vi "FTP Move files.vi"(0 "File Management":T2, 1 "Unmanaged Files Queue":refnum<queue>, 3 "FTP Creds":T1 {"FTP Timeout (S)" min=0 max=300 step=1}, 4 "File output directories":T3={"Archive Location"=path "", "Archive Location 2"=path "<Not A Path>", "OutPut Path"=path "", "Directory(s) To Scan Files"=[]}, 5 "Unmanaged Files prior errors":errorcluster, 6 "Timing true or false to zip files":bool) -> (15 "Unmanaged Files Queue out":refnum<queue>, 16 "Unmanaged files queue error out":errorcluster, 19 "Log file write error condition":errorcluster)   [LabVIEW 2011]
uses:
  Controls/File Path directories.ctl
  Controls/File Management.ctl
  Controls/FTP Credintials.ctl
  <vilib>/Utility/sysdir.llb/System Directory Type.ctl
panel:
  # "File Handling Method"
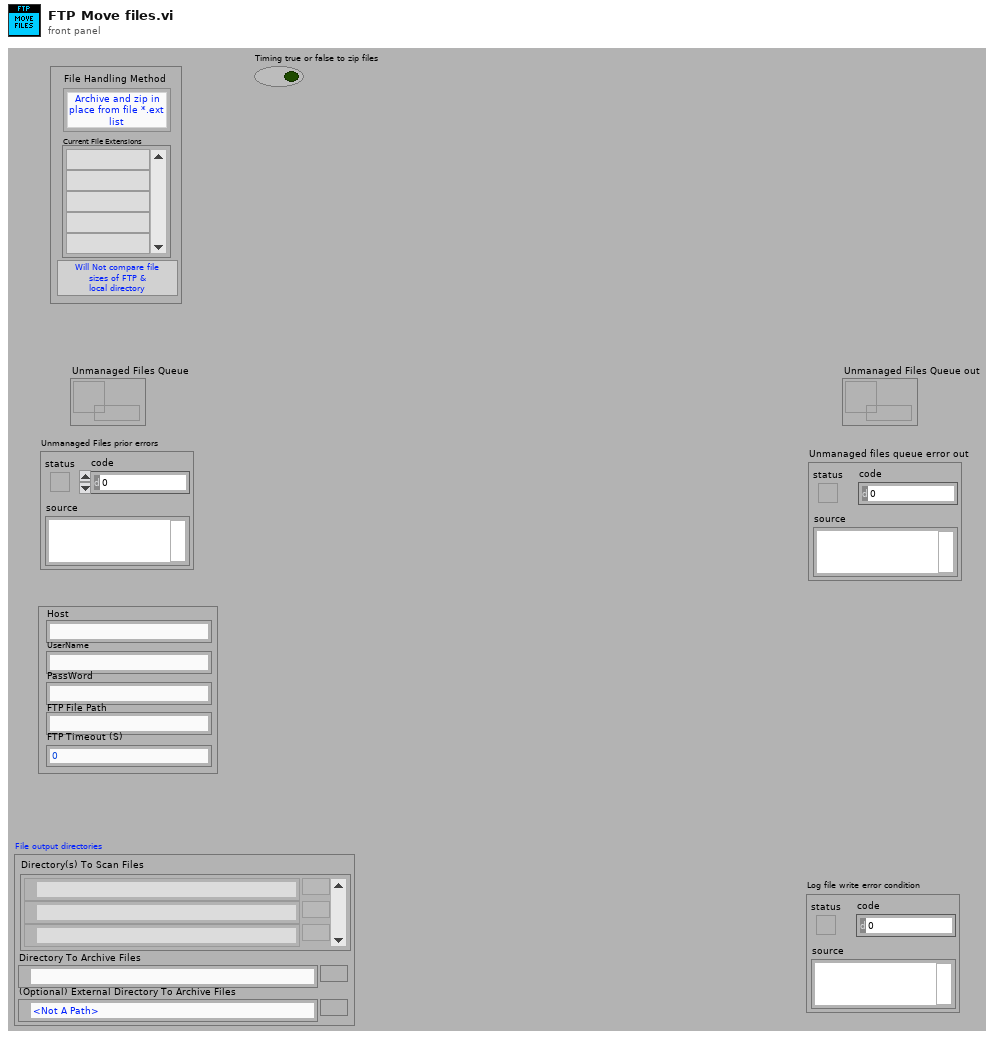
[diagram p1: front panel]
types:
  T1 = typedef "FTP Credintials.ctl" = cluster{"Host":string, "UserName":string, "PassWord":string, "FTP File Path":string, "FTP Timeout (S)":i32, "Active or Passive":bool, "ASCII or Binary":bool}
  T2 = typedef "File Management.ctl" = cluster{"Comp File Size":bool, "File Handle Method":enum16{"Archive and zip in place from file *.ext list", "Archive and zip ALL file Types to archive directory", "Archive and zip to archive directory from file *.ext list", "Perform no file management"}, "file extention list":string[]}
  T3 = typedef "File Path directories.ctl" = cluster{"Archive Location":path, "Archive Location 2":path, "OutPut Path":path, "Directory(s) To Scan Files":path[]}
  T4 = enum16{"Archive and zip in place from file *.ext list", "Archive and zip ALL file Types to archive directory", "Archive and zip to archive directory from file *.ext list", "Perform no file management"}
  T5 = typedef "System Directory Type.ctl" = i32
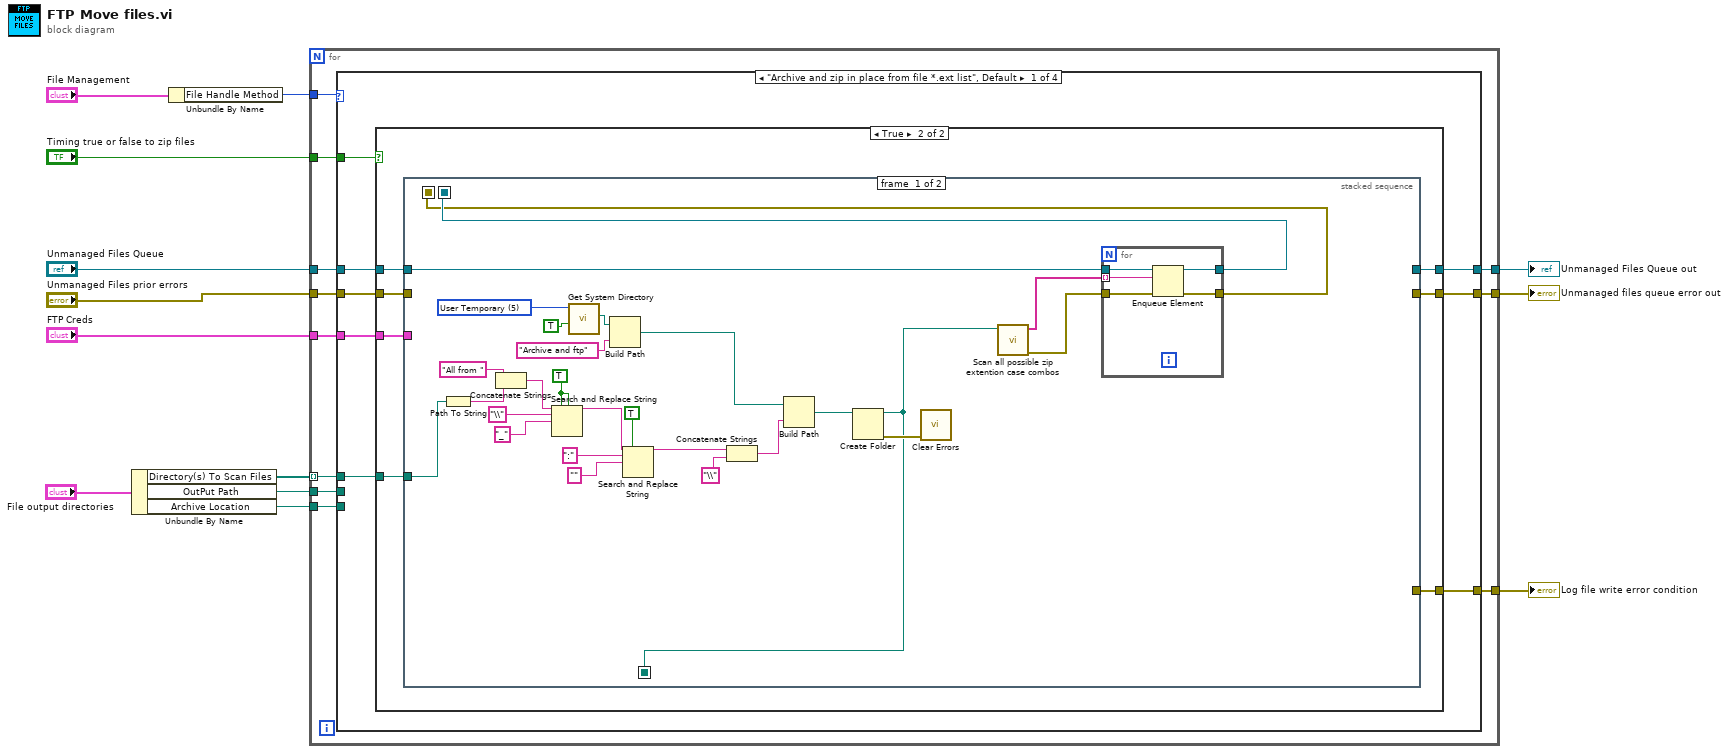
[diagram p0: block diagram]
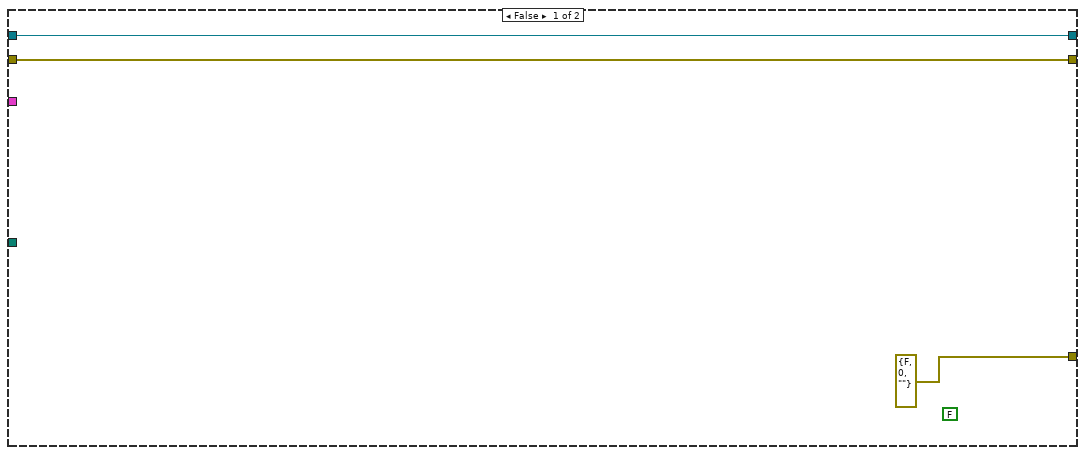
[diagram p2: hidden frame]
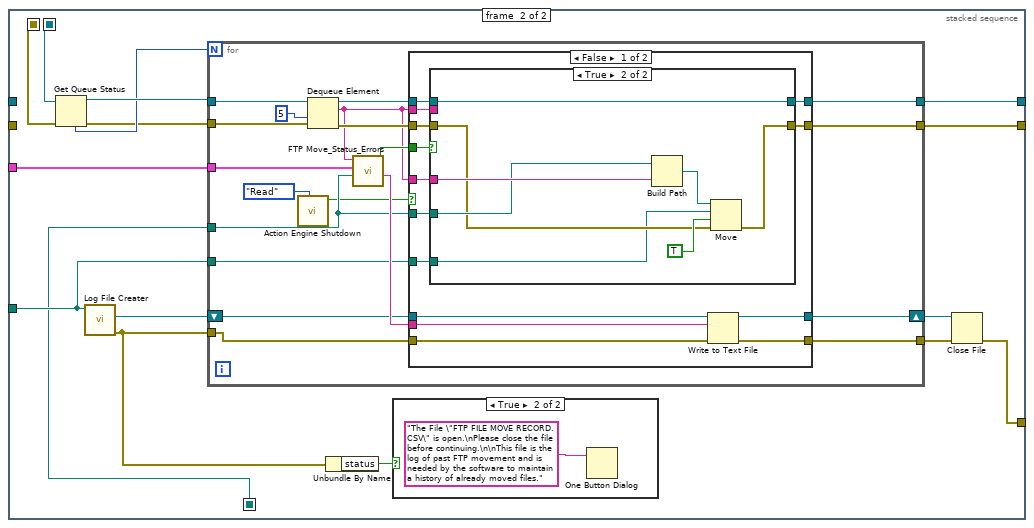
[diagram p3: hidden frame]
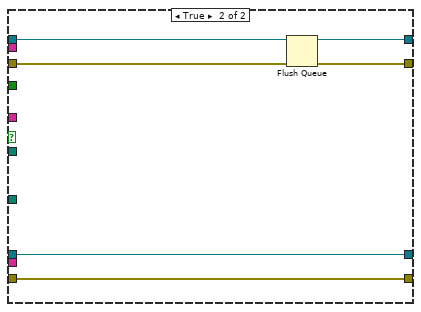
[diagram p6: hidden frame]
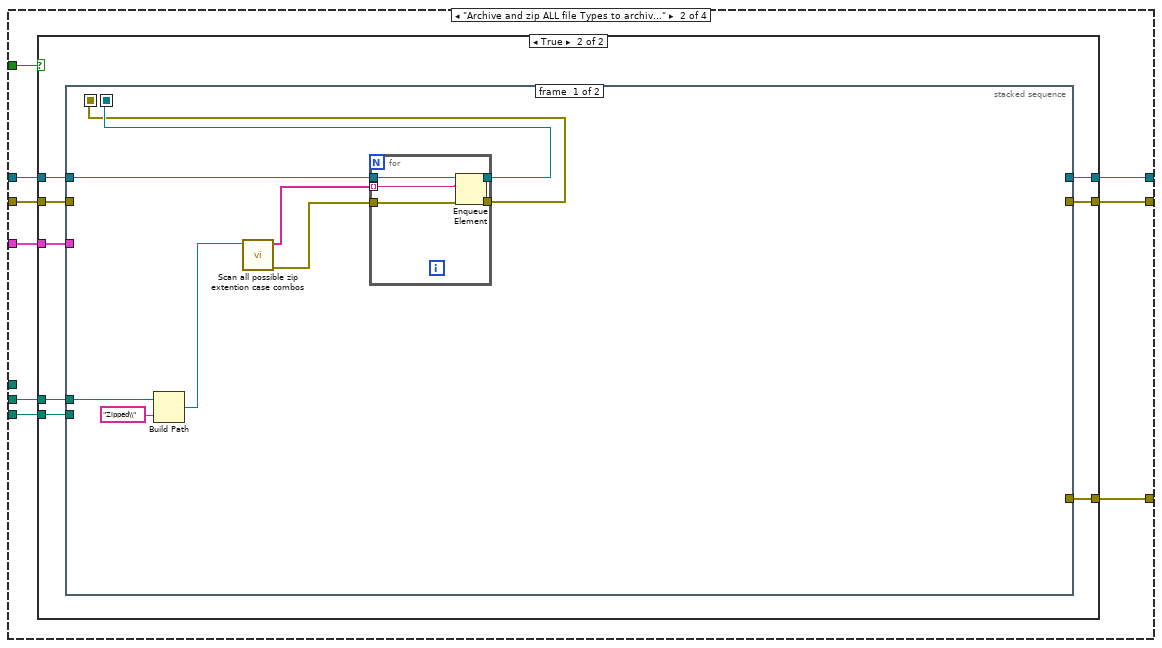
[diagram p7: hidden frame]
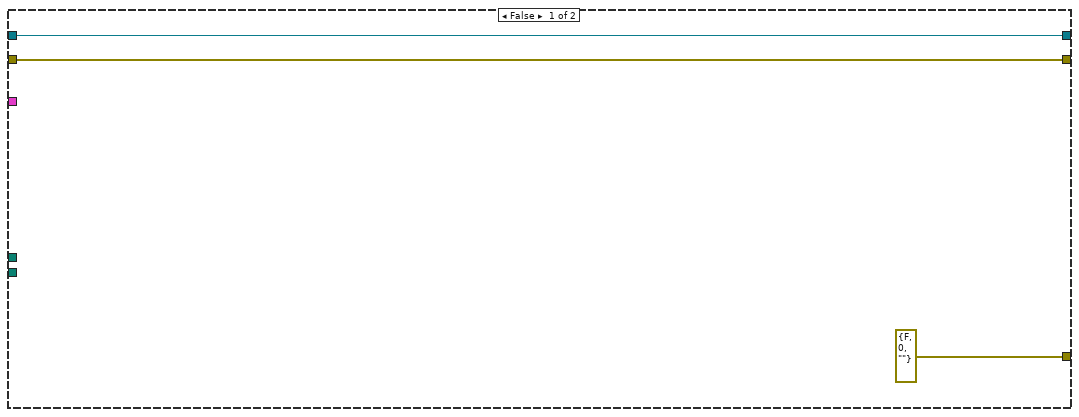
[diagram p8: hidden frame]
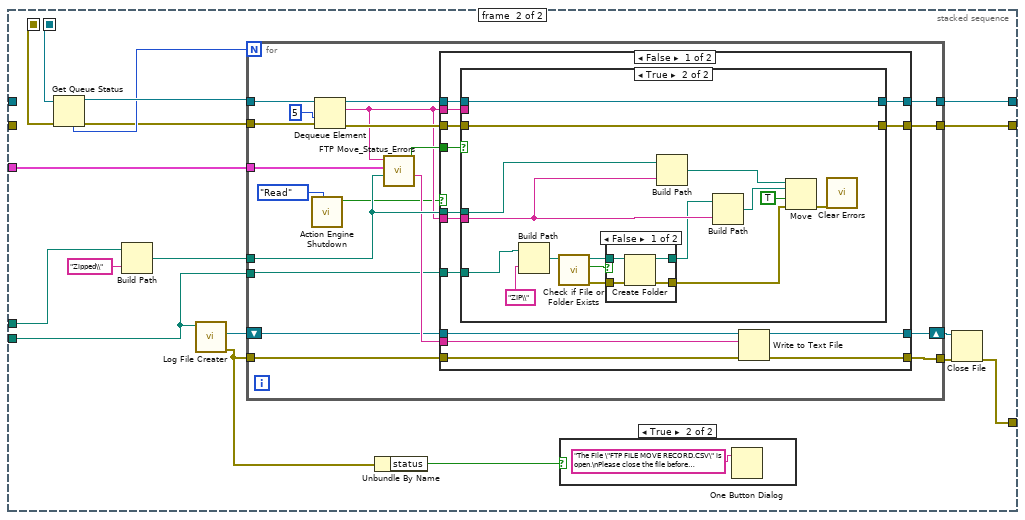
[diagram p9: hidden frame]
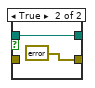
[diagram p12: hidden frame]
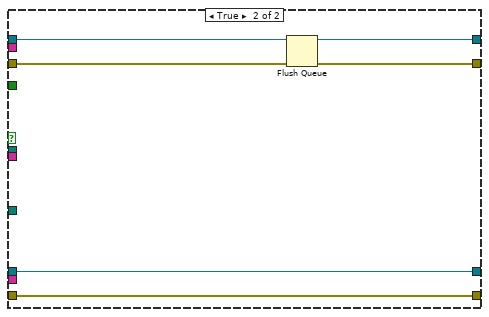
[diagram p13: hidden frame]
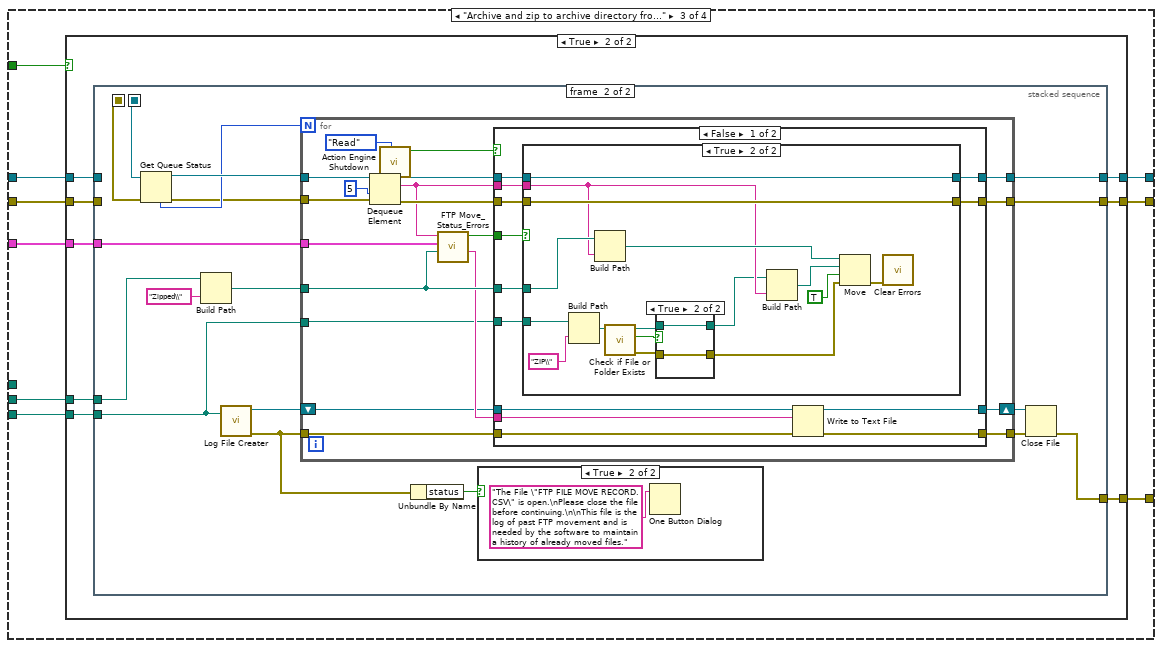
[diagram p14: hidden frame]
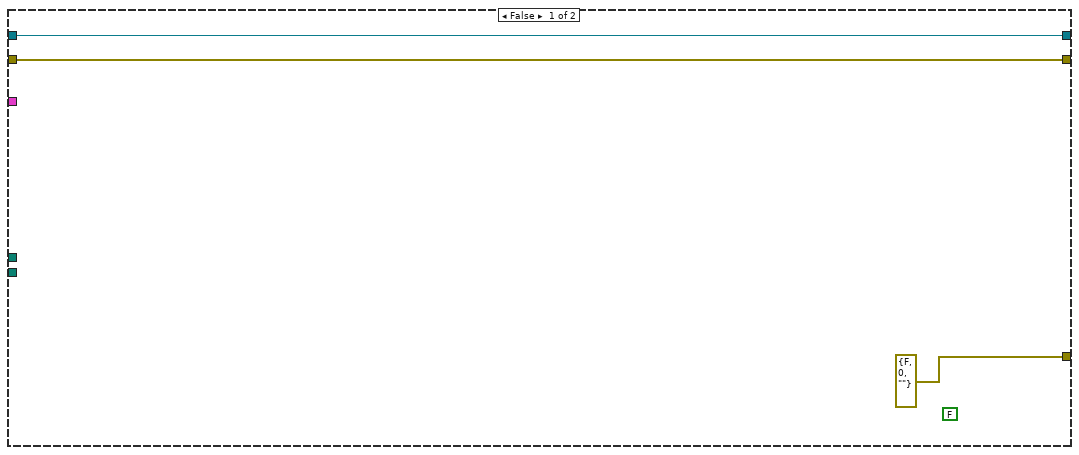
[diagram p15: hidden frame]
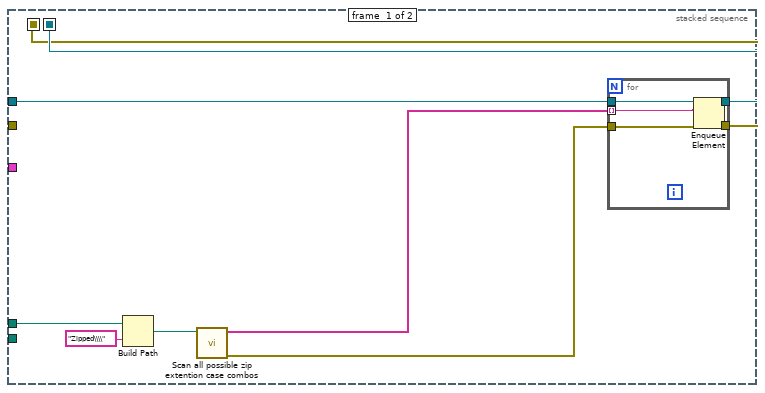
[diagram p16: hidden frame]
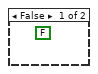
[diagram p17: hidden frame]
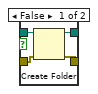
[diagram p19: hidden frame]
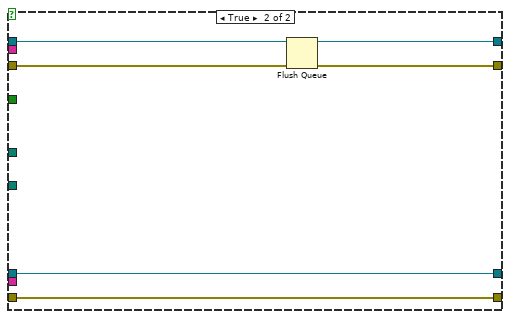
[diagram p20: hidden frame]
diagram:
  n1 = Unbundle By Name("File output directories") -> ("Directory(s) To Scan Files"=w1:path[], "OutPut Path"=w4:path, "Archive Location"=w3:path)
  n2 = Unbundle By Name("File Management") -> ("File Handle Method"=w5:T4)
  n3 = for {
    tunnel: "Unmanaged Files Queue" -> [w24]
    tunnel: "Unmanaged Files prior errors" -> [w23]
    tunnel: "Timing true or false to zip files" -> [w22]
    tunnel: [w21] -> w10
    tunnel: [w20] -> w9
    tunnel: [w19] -> w8
    tunnel: w5 -> [w18]
    tunnel: w4 -> [w17]
    tunnel: w3 -> [w16]
    tunnel: "FTP Creds" -> [w15]
    tunnel: w1 -> [w14] mode=indexing
    n4 = case shown="\"Archive and zip in place from file *.ext list\", Default" w18 {
      tunnel: w24 -> [w31 w149 w263 w372]
      tunnel: w23 -> [w30 w148 w262 w371]
      tunnel: w15 -> [w29 w147 w261 _]
      tunnel: w17 -> [_ w146 w260 _]
      tunnel: w22 -> [w32 w145 w264 _]
      tunnel: [w27 w144 w258 w372] -> w21
      tunnel: [w26 w143 w257 w371] -> w20
      tunnel: [w25 w142 w256 errorcluster {"status"=FALSE, "code"=0, "source"=""} ("error out")] -> w19
      tunnel: w16 -> [_ w141 w259 _]
      tunnel: w14 -> [w28 _ _ _]
      frame "Archive and zip in place from file *.ext list", Default {
        n5 = case shown="True" w32 {
          tunnel: w31 -> [w35 w42]
          tunnel: [w35 w41] -> w27
          tunnel: w30 -> [w34 w40]
          tunnel: [w34 w39] -> w26
          tunnel: [errorcluster {"status"=FALSE, "code"=0, "source"=""} ("error out") w36] -> w25
          tunnel: w29 -> [_ w38]
          tunnel: w28 -> [_ w37]
          frame False {
            (unwired) FALSE
          }
          frame True {
            n6 = stacked-sequence {
              seq-local: [w68 _] -> [_ w89]
              seq-local: [w67 _] -> [_ w83]
              seq-local: [w45 _] -> [_ w76]
              tunnel: w42 -> [w69 _]
              tunnel: [_ w90] -> w41
              tunnel: w40 -> [_ _]
              tunnel: [_ w85] -> w39
              tunnel: w38 -> [_ w84]
              tunnel: w37 -> [w46 w77]
              tunnel: [_ w80] -> w36
              frame #0 {
                w57 = TRUE ("replace all? (F)")
                w50 = T5 5 items=["User Home"=0, "User Desktop"=1, "User Documents"=2, "User Application Data"=3, "User Preferences"=4, "User Temporary"=5, "Public Documents"=6, "Public Application Data"=7, "Public Preferences"=8, "Public Cache"=13, "System Core Libraries"=9, "System Installed Libraries"=10, "Application Files"=11, "Boot Volume Root"=12] ("system directory type")
                n7 = Path To String(path=w46) -> (string=w53:string)
                n8 = Concatenate Strings("All from " ("name or relative path"), w53) -> (w54:string)
                n9 = Search and Replace String(replace all?=w57, case sensitive?=w57, input string=w54, search string="\\" ("replace string (\"\")"), replace string="_" ("replace string (\"\")")) -> (result string=w60:string)  [unwired: 3 in, 3 out]
                n10 = call <vilib>:"Get System Directory.vi"("create directory if not found? (F)"=TRUE, "system directory type"=w50) -> ("system directory"=w48:path)  [unwired: 9 in]
                n11 = Build Path(base path=w48, name or relative path="Archive and ftp") -> (appended path=w62:path)
                n12 = Search and Replace String(replace all?=TRUE ("replace all? (F)"), input string=w60, search string=":" ("replace string (\"\")"), replace string="" ("replace string (\"\")")) -> (result string=w63:string)  [unwired: 4 in, 3 out]
                n13 = Concatenate Strings(w63, "\\" ("replace string (\"\")")) -> (w65:string)
                n14 = Build Path(base path=w62, name or relative path=w65) -> (appended path=w66:path)
                n15 = Create Folder(path (use dialog)=w66) -> (created path=w45:path, error out=w51:errorcluster)  [unwired: 2 in, 1 out]
                n16 = call <vilib>:"Clear Errors.vi"("error in (no error)"=w51) -> ()  [unwired: 6 in, 1 out]
                n17 = call "Scan all possible zip extention case combos.vi"("Path containing Zipped files"=w45) -> ("error out"=w43:errorcluster, "Zipped Files List"=w44:string[])  [unwired: 9 in]
                n18 = for {
                  tunnel: w69 -> [w74]
                  tunnel: [w73] -> w67
                  tunnel: [w72] -> w68
                  tunnel: w44 -> [w71] mode=indexing
                  tunnel: w43 -> [w70]
                  n19 = Enqueue Element(queue=w74, element=w71, error in (no error)=w70) -> (queue out=w72:refnum<queue>, error out=w73:errorcluster)  [unwired: 1 in, 1 out]
                }
              }
              frame #1 {
                n20 = Get Queue Status(queue=w89, error in (no error)=w83) -> (queue out=w88:refnum<queue>, error out=w86:errorcluster, # elements in queue=w87:i32)  [unwired: 1 in, 5 out]
                n21 = call "Log File Creater.vi"("FTP log file path"=w77) -> ("all condition error"=w75:errorcluster, "File Refnum"=w79:refnum<file>)  [unwired: 8 in, 1 out]
                n22 = for {
                  N: w87 -> [_]
                  tunnel: w88 -> [w103]
                  tunnel: [w109] -> w90
                  tunnel: w86 -> [w102]
                  tunnel: [w106] -> w85
                  tunnel: w84 -> [w105]
                  tunnel: w77 -> [w99]
                  tunnel: w76 -> [w98]
                  tunnel: [w96] -> w81
                  tunnel: w75 -> [w94]
                  shift-right: [w97] -> w78
                  shift-left: w79 -> [w95]
                  n23 = call "Action Engine Shutdown.vi"("Shutdown"=enum16{"Write", "Read"}."Read") -> ("Shutdown"=w92:bool)  [unwired: 9 in, 1 out]
                  n24 = Dequeue Element(queue=w103, timeout in ms (-1)=5, error in (no error)=w102) -> (queue out=w110:refnum<queue>, element=w100:string, error out=w107:errorcluster)  [unwired: 1 out]
                  n25 = call "FTP Move_Status_Errors.vi"("Dir of file to FTP"=w98, "FTP input cluster"=w105, "File to Move"=w100) -> ("concatenated string of Error"=w101:string, "FTP completed (true = good)"=w104:bool)  [unwired: 7 in]
                  n26 = case shown="False" w92 {
                    tunnel: [w124 w136] -> w97
                    tunnel: [w123 w135] -> w96
                    tunnel: w110 -> [w122 w140]
                    tunnel: [w121 w139] -> w109
                    tunnel: w107 -> [w120 w138]
                    tunnel: [w119 w137] -> w106
                    tunnel: w101 -> [w118 _]
                    tunnel: w104 -> [w117 _]
                    tunnel: w100 -> [w116 _]
                    tunnel: w99 -> [w115 _]
                    tunnel: w100 -> [w114 _]
                    tunnel: w95 -> [w113 w136]
                    tunnel: w94 -> [w112 w135]
                    tunnel: w98 -> [w111 _]
                    frame False {
                      n27 = case shown="True" w117 {
                        tunnel: w122 -> [w126 w134]
                        tunnel: w116 -> [_ _]
                        tunnel: [w126 w134] -> w121
                        tunnel: w120 -> [w125 w128]
                        tunnel: [w125 w131] -> w119
                        tunnel: w115 -> [_ w127]
                        tunnel: w114 -> [_ w133]
                        tunnel: w111 -> [_ w129]
                        frame False {
                          # "If Error occurs in ftp then leave element alone\nand it will be requeued next time process runs."
                        }
                        frame True {
                          n28 = Build Path(base path=w129, name or relative path=w133) -> (appended path=w132:path)
                          n29 = Move(source path=w132, error in=w128, 9:TRUE ("overwrite (F)"), 10:w127) -> (error out=w131:errorcluster)  [unwired: 1 in, 2 out]
                        }
                      }
                      n30 = Write to Text File(file (use dialog)=w113, text=w118, error in=w112) -> (refnum out=w124:refnum<file>, error out=w123:errorcluster)  [unwired: 1 in, 1 out]
                    }
                    frame True {
                      n31 = Flush Queue(queue=w140, error in (no error)=w138) -> (queue out=w139:refnum<queue>, error out=w137:errorcluster)  [unwired: 1 out]
                    }
                  }
                }
                n32 = Unbundle By Name(w75) -> ("status"=w82:bool)
                n33 = case shown="True" w82 {
                  frame False {
                  }
                  frame True {
                    n34 = One Button Dialog(message="The File \"FTP FILE MOVE RECORD.CSV\" is open.\nPlease close the file before continuing.\n\nThis file is the log of past FTP movement and is needed by the software to maintain a history of already moved files.") -> ()  [unwired: 1 in, 1 out]
                  }
                }
                n35 = Close File(refnum=w78, error in=w81) -> (error out=w80:errorcluster)  [unwired: 1 out]
              }
            }
          }
        }
      }
      frame "Archive and zip ALL file Types to archive directory" {
        n36 = case shown="True" w145 {
          tunnel: w149 -> [w152 w160]
          tunnel: [w152 w159] -> w144
          tunnel: w148 -> [w151 w158]
          tunnel: [w151 w157] -> w143
          tunnel: [errorcluster {"status"=FALSE, "code"=0, "source"=""} ("error out") w153] -> w142
          tunnel: w147 -> [_ w156]
          tunnel: w146 -> [_ w155]
          tunnel: w141 -> [_ w154]
          frame False {
          }
          frame True {
            n37 = stacked-sequence {
              seq-local: [w167 _] -> [_ w190]
              seq-local: [w166 _] -> [_ w184]
              tunnel: w160 -> [w168 _]
              tunnel: [_ w191] -> w159
              tunnel: w158 -> [_ _]
              tunnel: [_ w186] -> w157
              tunnel: w156 -> [_ w185]
              tunnel: w155 -> [w165 w175]
              tunnel: w154 -> [_ w178]
              tunnel: [_ w180] -> w153
              frame #0 {
                n38 = Build Path(base path=w165, name or relative path="Zipped\\") -> (appended path=w163:path)
                n39 = call "Scan all possible zip extention case combos.vi"("Path containing Zipped files"=w163) -> ("error out"=w161:errorcluster, "Zipped Files List"=w162:string[])  [unwired: 9 in]
                n40 = for {
                  tunnel: w168 -> [w173]
                  tunnel: [w172] -> w166
                  tunnel: [w171] -> w167
                  tunnel: w162 -> [w170] mode=indexing
                  tunnel: w161 -> [w169]
                  n41 = Enqueue Element(queue=w173, element=w170, error in (no error)=w169) -> (queue out=w171:refnum<queue>, error out=w172:errorcluster)  [unwired: 1 in, 1 out]
                }
              }
              frame #1 {
                n42 = Get Queue Status(queue=w190, error in (no error)=w184) -> (queue out=w189:refnum<queue>, error out=w187:errorcluster, # elements in queue=w188:i32)  [unwired: 1 in, 5 out]
                n43 = Build Path(base path=w175, name or relative path="Zipped\\") -> (appended path=w176:path)
                n44 = call "Log File Creater.vi"("FTP log file path"=w178) -> ("all condition error"=w174:errorcluster, "File Refnum"=w179:refnum<file>)  [unwired: 8 in, 1 out]
                n45 = for {
                  N: w188 -> [_]
                  tunnel: w189 -> [w204]
                  tunnel: [w210] -> w191
                  tunnel: w187 -> [w203]
                  tunnel: [w207] -> w186
                  tunnel: w185 -> [w206]
                  tunnel: w176 -> [w202]
                  tunnel: [w198] -> w181
                  tunnel: w174 -> [w196]
                  tunnel: w178 -> [w195]
                  shift-right: [w199] -> w182
                  shift-left: w179 -> [w197]
                  n46 = call "Action Engine Shutdown.vi"("Shutdown"=enum16{"Write", "Read"}."Read") -> ("Shutdown"=w193:bool)  [unwired: 9 in, 1 out]
                  n47 = Dequeue Element(queue=w204, timeout in ms (-1)=5, error in (no error)=w203) -> (queue out=w211:refnum<queue>, element=w200:string, error out=w208:errorcluster)  [unwired: 1 out]
                  n48 = call "FTP Move_Status_Errors.vi"("Dir of file to FTP"=w202, "FTP input cluster"=w206, "File to Move"=w200) -> ("concatenated string of Error"=w201:string, "FTP completed (true = good)"=w205:bool)  [unwired: 7 in]
                  n49 = case shown="False" w193 {
                    tunnel: [w225 w251] -> w199
                    tunnel: [w224 w250] -> w198
                    tunnel: w211 -> [w223 w255]
                    tunnel: [w222 w254] -> w210
                    tunnel: w208 -> [w221 w253]
                    tunnel: [w220 w252] -> w207
                    tunnel: w201 -> [w219 _]
                    tunnel: w205 -> [w218 _]
                    tunnel: w200 -> [w217 _]
                    tunnel: w202 -> [w216 _]
                    tunnel: w200 -> [w215 _]
                    tunnel: w197 -> [w214 w251]
                    tunnel: w196 -> [w213 w250]
                    tunnel: w195 -> [w212 _]
                    frame False {
                      n50 = case shown="True" w218 {
                        tunnel: w223 -> [w227 w243]
                        tunnel: w217 -> [_ _]
                        tunnel: [w227 w243] -> w222
                        tunnel: w221 -> [w226 w242]
                        tunnel: [w226 w242] -> w220
                        tunnel: w216 -> [_ w241]
                        tunnel: w215 -> [_ w238]
                        tunnel: w212 -> [_ w231]
                        frame False {
                        }
                        frame True {
                          n51 = Build Path(base path=w231, name or relative path="ZIP\\") -> (appended path=w234:path)
                          n52 = call <vilib>:"Check if File or Folder Exists.vi"("path"=w234) -> ("error out"=w228:errorcluster, "file or folder exists?"=w235:bool, "dup path"=w236:path)  [unwired: 8 in]
                          n53 = case shown="False" w235 {
                            tunnel: w236 -> [w247 w249]
                            tunnel: [w246 w249] -> w232
                            tunnel: [w245 errorcluster {"status"=FALSE, "code"=0, "source"=""} ("error out")] -> w230
                            tunnel: w228 -> [w244 _]
                            frame False {
                              n54 = Create Folder(path (use dialog)=w247, error in=w244) -> (created path=w246:path, error out=w245:errorcluster)  [unwired: 1 in, 1 out]
                            }
                            frame True {
                            }
                          }
                          n55 = Build Path(base path=w241, name or relative path=w238) -> (appended path=w240:path)
                          n56 = Build Path(base path=w232, name or relative path=w238) -> (appended path=w239:path)
                          n57 = Move(source path=w240, error in=w230, 9:TRUE ("overwrite (F)"), 10:w239) -> (error out=w229:errorcluster)  [unwired: 1 in, 2 out]
                          n58 = call <vilib>:"Clear Errors.vi"("error in (no error)"=w229) -> ()  [unwired: 6 in, 1 out]
                        }
                      }
                      n59 = Write to Text File(file (use dialog)=w214, text=w219, error in=w213) -> (refnum out=w225:refnum<file>, error out=w224:errorcluster)  [unwired: 1 in, 1 out]
                    }
                    frame True {
                      n60 = Flush Queue(queue=w255, error in (no error)=w253) -> (queue out=w254:refnum<queue>, error out=w252:errorcluster)  [unwired: 1 out]
                    }
                  }
                }
                n61 = Unbundle By Name(w174) -> ("status"=w183:bool)
                n62 = case shown="True" w183 {
                  frame False {
                  }
                  frame True {
                    n63 = One Button Dialog(message="The File \"FTP FILE MOVE RECORD.CSV\" is open.\nPlease close the file before continuing.\n\nThis file is the log of past FTP movement and is needed by the software to maintain a history of already moved files.") -> ()  [unwired: 1 in, 1 out]
                  }
                }
                n64 = Close File(refnum=w182, error in=w181) -> (error out=w180:errorcluster)  [unwired: 1 out]
              }
            }
          }
        }
      }
      frame "Archive and zip to archive directory from file *.ext list" {
        n65 = case shown="True" w264 {
          tunnel: w263 -> [w267 w275]
          tunnel: [w267 w274] -> w258
          tunnel: w262 -> [w266 w273]
          tunnel: [w266 w272] -> w257
          tunnel: [errorcluster {"status"=FALSE, "code"=0, "source"=""} ("error out") w271] -> w256
          tunnel: w261 -> [_ w270]
          tunnel: w260 -> [_ w269]
          tunnel: w259 -> [_ w268]
          frame False {
            (unwired) FALSE
          }
          frame True {
            n66 = stacked-sequence {
              seq-local: [w282 _] -> [_ w305]
              seq-local: [w279 _] -> [_ w299]
              tunnel: w275 -> [w283 _]
              tunnel: [_ w306] -> w274
              tunnel: w273 -> [_ _]
              tunnel: [_ w301] -> w272
              tunnel: [_ w295] -> w271
              tunnel: w270 -> [_ w300]
              tunnel: w269 -> [w278 w290]
              tunnel: w268 -> [_ w293]
              frame #0 {
                n67 = Build Path(base path=w278, name or relative path="Zipped\\\\") -> (appended path=w277:path)
                n68 = call "Scan all possible zip extention case combos.vi"("Path containing Zipped files"=w277) -> ("error out"=w280:errorcluster, "Zipped Files List"=w281:string[])  [unwired: 9 in]
                n69 = for {
                  tunnel: w283 -> [w288]
                  tunnel: [w287] -> w279
                  tunnel: [w286] -> w282
                  tunnel: w281 -> [w285] mode=indexing
                  tunnel: w280 -> [w284]
                  n70 = Enqueue Element(queue=w288, element=w285, error in (no error)=w284) -> (queue out=w286:refnum<queue>, error out=w287:errorcluster)  [unwired: 1 in, 1 out]
                }
              }
              frame #1 {
                n71 = Get Queue Status(queue=w305, error in (no error)=w299) -> (queue out=w304:refnum<queue>, error out=w302:errorcluster, # elements in queue=w303:i32)  [unwired: 1 in, 5 out]
                n72 = Build Path(base path=w290, name or relative path="Zipped\\") -> (appended path=w291:path)
                n73 = call "Log File Creater.vi"("FTP log file path"=w293) -> ("all condition error"=w289:errorcluster, "File Refnum"=w294:refnum<file>)  [unwired: 8 in, 1 out]
                n74 = for {
                  N: w303 -> [_]
                  tunnel: w304 -> [w319]
                  tunnel: [w325] -> w306
                  tunnel: [w313] -> w296
                  tunnel: w302 -> [w318]
                  tunnel: [w322] -> w301
                  tunnel: w300 -> [w321]
                  tunnel: w291 -> [w317]
                  tunnel: w293 -> [w312]
                  tunnel: w289 -> [w310]
                  shift-right: [w314] -> w297
                  shift-left: w294 -> [w311]
                  n75 = Dequeue Element(queue=w319, timeout in ms (-1)=5, error in (no error)=w318) -> (queue out=w326:refnum<queue>, element=w315:string, error out=w323:errorcluster)  [unwired: 1 out]
                  n76 = call "Action Engine Shutdown.vi"("Shutdown"=enum16{"Write", "Read"}."Read") -> ("Shutdown"=w308:bool)  [unwired: 9 in, 1 out]
                  n77 = call "FTP Move_Status_Errors.vi"("Dir of file to FTP"=w317, "FTP input cluster"=w321, "File to Move"=w315) -> ("concatenated string of Error"=w316:string, "FTP completed (true = good)"=w320:bool)  [unwired: 7 in]
                  n78 = case shown="False" w308 {
                    tunnel: [w339 w365] -> w314
                    tunnel: [w338 w364] -> w313
                    tunnel: w326 -> [w337 w369]
                    tunnel: [w336 w368] -> w325
                    tunnel: w323 -> [w335 w367]
                    tunnel: [w334 w366] -> w322
                    tunnel: w316 -> [w333 _]
                    tunnel: w320 -> [w332 _]
                    tunnel: w317 -> [w331 _]
                    tunnel: w315 -> [w330 _]
                    tunnel: w311 -> [w329 w365]
                    tunnel: w310 -> [w328 w364]
                    tunnel: w312 -> [w327 _]
                    frame False {
                      n79 = case shown="True" w332 {
                        tunnel: w337 -> [w341 w357]
                        tunnel: [w341 w357] -> w336
                        tunnel: w335 -> [w340 w356]
                        tunnel: [w340 w356] -> w334
                        tunnel: w331 -> [_ w355]
                        tunnel: w330 -> [_ w352]
                        tunnel: w327 -> [_ w345]
                        frame False {
                        }
                        frame True {
                          n80 = Build Path(base path=w345, name or relative path="ZIP\\") -> (appended path=w348:path)
                          n81 = Build Path(base path=w355, name or relative path=w352) -> (appended path=w354:path)
                          n82 = call <vilib>:"Check if File or Folder Exists.vi"("path"=w348) -> ("error out"=w344:errorcluster, "file or folder exists?"=w349:bool, "dup path"=w350:path)  [unwired: 8 in]
                          n83 = case shown="True" w349 {
                            tunnel: w350 -> [w361 w363]
                            tunnel: [w360 w363] -> w346
                            tunnel: w344 -> [w359 w362]
                            tunnel: [w358 w362] -> w343
                            frame False {
                              n84 = Create Folder(path (use dialog)=w361, error in=w359) -> (created path=w360:path, error out=w358:errorcluster)  [unwired: 1 in, 1 out]
                            }
                            frame True {
                            }
                          }
                          n85 = Build Path(base path=w346, name or relative path=w352) -> (appended path=w353:path)
                          n86 = Move(source path=w354, error in=w343, 9:TRUE ("overwrite (F)"), 10:w353) -> (error out=w342:errorcluster)  [unwired: 1 in, 2 out]
                          n87 = call <vilib>:"Clear Errors.vi"("error in (no error)"=w342) -> ()  [unwired: 6 in, 1 out]
                        }
                      }
                      n88 = Write to Text File(file (use dialog)=w329, text=w333, error in=w328) -> (refnum out=w339:refnum<file>, error out=w338:errorcluster)  [unwired: 1 in, 1 out]
                    }
                    frame True {
                      n89 = Flush Queue(queue=w369, error in (no error)=w367) -> (queue out=w368:refnum<queue>, error out=w366:errorcluster)  [unwired: 1 out]
                    }
                  }
                }
                n90 = Unbundle By Name(w289) -> ("status"=w298:bool)
                n91 = case shown="True" w298 {
                  frame False {
                    (unwired) FALSE
                  }
                  frame True {
                    n92 = One Button Dialog(message="The File \"FTP FILE MOVE RECORD.CSV\" is open.\nPlease close the file before continuing.\n\nThis file is the log of past FTP movement and is needed by the software to maintain a history of already moved files.") -> ()  [unwired: 1 in, 1 out]
                  }
                }
                n93 = Close File(refnum=w297, error in=w296) -> (error out=w295:errorcluster)  [unwired: 1 out]
              }
            }
          }
        }
      }
      frame "Perform no file management" {
      }
    }
  }
  "Unmanaged Files Queue out" <- w10
  "Unmanaged files queue error out" <- w9
  "Log file write error condition" <- w8
